vi "Process Data.vi"(6 "dt":dbl, 8 "error in (no error)":errorcluster, 9 "t0":dbl, 10 "Data":dbl[][](array[numeric]), 11 "DataLogger in":refnum<class "DataLogger.lvclass">) -> (0 "error out":errorcluster, 3 "DataLogger out":refnum<class "DataLogger.lvclass">)   [LabVIEW 2020, in "VolatusData.lvlib" / "DataLogger.lvclass"]
uses:
  DataLogger.lvclass
  DataLogger.lvclass/DataLogger.ctl
  Volatus/Task/Task.lvclass
  C:/dev/lv20CE/relink/lv-volatus/VolatusData/DataHandlerTask/DataHandlerTask.lvclass
  C:/dev/lv20CE/relink/lv-volatus/Volatus/Task/Task.lvclass
  C:/Program Files (x86)/National Instruments/LabVIEW 2020/vi.lib/ActorFramework/Actor/Actor.lvclass
  C:/dev/lv20CE/relink/lv-volatus/Volatus/TaskStateHandler/TaskStateHandler.lvclass
  C:/dev/lv20CE/relink/lv-volatus/Volatus/VectoMessageHandler/VectoMessageHandler.lvclass
  C:/dev/lv20CE/relink/lv-volatus/Volatus/API Provider/API Provider.lvclass
  C:/dev/lv20CE/relink/lv-volatus/VolatusData/DataHandler/DataHandler.lvclass
  C:/dev/lv20CE/relink/lv-volatus/VolatusData/DataLogger/DataLogger.lvclass
  C:/dev/lv20CE/relink/lv-volatus/VolatusData/LoggingHandler/LoggingHandler.lvclass
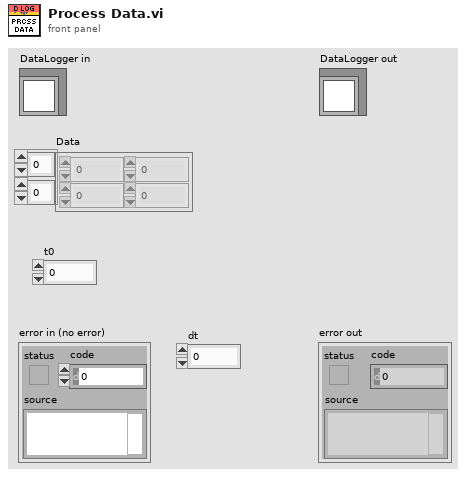
[diagram p1: front panel]
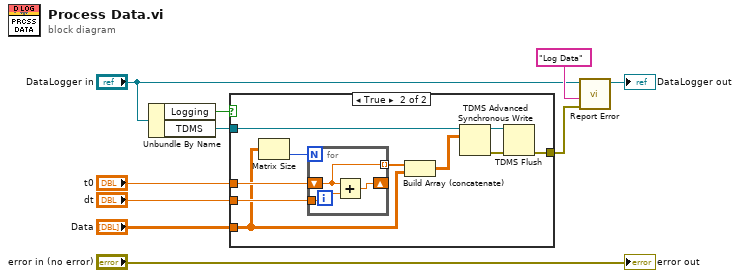
[diagram p0: block diagram]
diagram:
  n1 = Unbundle By Name("DataLogger in") -> ("Logging"=w9:bool, "TDMS"=w8:refnum<k34>)
  n2 = case shown="True" w9 {
    tunnel: "Data" -> [_ w13]
    tunnel: "t0" -> [_ w20]
    tunnel: "dt" -> [_ w19]
    tunnel: w8 -> [_ w17]
    tunnel: [_ w14] -> w7
    frame False {
    }
    frame True {
      n3 = Matrix Size(0:w13) -> (2:w12:i32)  [unwired: 1 out]
      n4 = for {
        N: w12 -> [_]
        tunnel: w19 -> [w23]
        shift-right: [w22] -> _
        shift-left: w20 -> [w21]
        tunnel: [w21] -> w18 mode=indexing
        n5 = Add(x=w21, y=w23) -> (x+y=w22:dbl)
      }
      n6 = Build Array (concatenate)(w18, w13) -> (w11:dbl[][])
      n7 = TDMS Advanced Synchronous Write(10:w11, 11:w17) -> (0:w15:errorcluster, 3:w16:refnum<k34>)  [unwired: 1 in]
      n8 = TDMS Flush(4:w15, 7:w16) -> (0:w14:errorcluster)  [unwired: 1 out]
    }
  }
  n9 = call "Report Error.vi"("error in (no error)"=w7, "Message"="Log Data", "Task in"="DataLogger in") -> ("Task out"=→"DataLogger out":refnum<class "DataLogger.lvclass">)  [unwired: 7 in, 1 out]
  "error out" <- "error in (no error)"
